vi "Set Direction.vi"(10 "Direction":bool, 11 "Reference in":T1) -> (3 "Reference out":T1)   [LabVIEW 2016, in "Impulse Data.lvclass"]
uses:
  Impulse Data.lvclass
  Instance handle.ctl
  Impulse Data.lvclass/Impulse Data.ctl
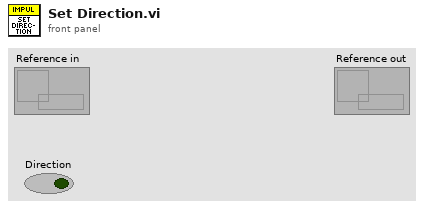
[diagram p1: front panel]
types:
  T1 = typedef "Impulse Data.lvclass/Instance handle.ctl" = refnum<data-value>
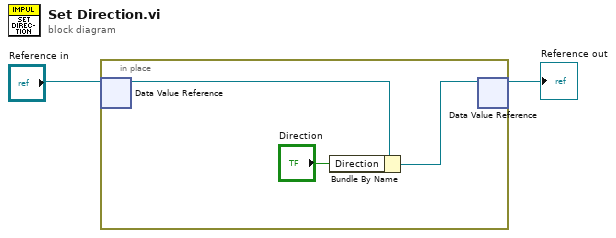
[diagram p0: block diagram]
diagram:
  n1 = in-place {
    n2 = in-place-dvr #1("Reference in") -> (w5:refnum<class "Impulse Data.lvclass">)  [unwired: 1 out]
    n3 = Bundle By Name(cluster=w5, "Direction"="Direction") -> (w4:refnum<class "Impulse Data.lvclass">)
    n4 = in-place-dvr #1(w4) -> (→"Reference out":T1)  [unwired: 1 out]
  }
